vi "UUID.vi"() -> (0 "UUID":string)   [LabVIEW 2018]
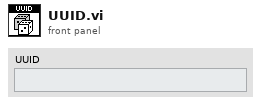
[diagram p1: front panel]
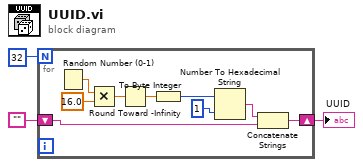
[diagram p0: block diagram]
diagram:
  n1 = for {
    N: 32 -> [_]
    shift-right: [w5] -> w1
    shift-left: "" -> [w4]
    n2 = Random Number (0-1)() -> (number: 0 to 1=w12:dbl)
    n3 = Multiply(x=w12, y=16.0) -> (x*y=w10:dbl)
    n4 = Round Toward -Infinity(1:w10) -> (0:w9:dbl)
    n5 = To Byte Integer(number=w9) -> (8bit integer=w8:i8)
    n6 = Number To Hexadecimal String(1:i16 1 ("width (-)"), 2:w8) -> (0:w6:string)
    n7 = Concatenate Strings(w6, w4) -> (w5:string)
  }
  "UUID" <- w1
